vi "train_data05_get.vi"(10 "文件路径（使用对话框）":path) -> (2 "数据":T1)   [LabVIEW 2014]
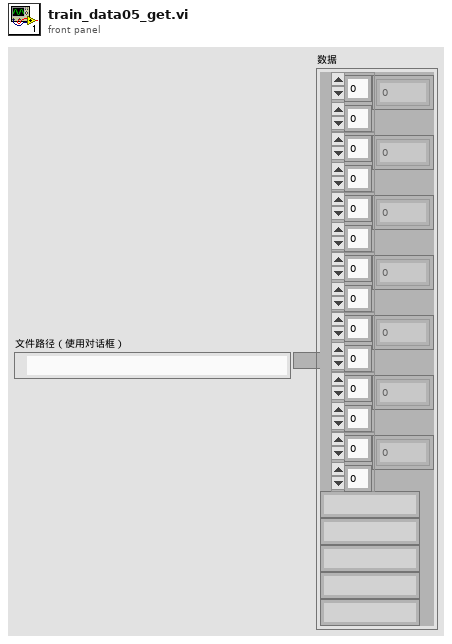
[diagram p1: front panel]
types:
  T1 = cluster{dbl[][], dbl[][], dbl[][], dbl[][], dbl[][], dbl[][], dbl[][], string, string, string, string, string}
  T2 = enum16{"open", "replace", "create", "open or create", "replace or create", "replace or create with confirmation"}
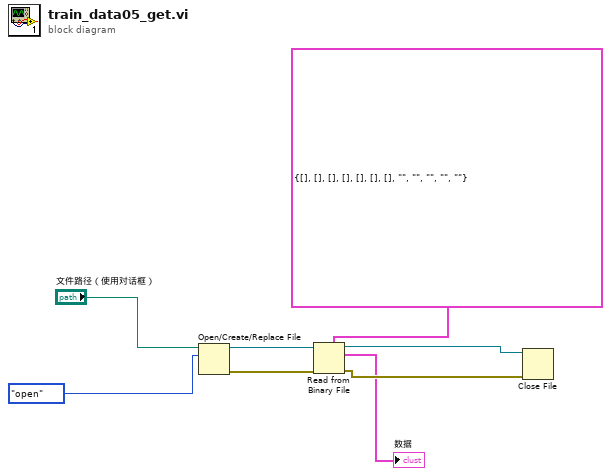
[diagram p0: block diagram]
diagram:
  n1 = Open/Create/Replace File(file path (use dialog)="文件路径（使用对话框）", operation (0:open)=T2."open") -> (refnum out=w8:refnum<file>, error out=w4:errorcluster)  [unwired: 4 in, 1 out]
  n2 = Read from Binary File(5:T1 {[], [], [], [], [], [], [], "", "", "", "", ""}, 8:w4, 11:w8) -> (0:w6:errorcluster, 2:→"数据":T1, 3:w5:refnum<file>)  [unwired: 3 in, 1 out]
  n3 = Close File(refnum=w5, error in=w6) -> ()  [unwired: 2 out]
